vi "Transport Delay (DBL).vi"(2 "initialize":bool, 3 "delay":i32, 4 "reset":bool, 5 "input point":dbl format="%.2f") -> (1 "output point":dbl format="%.2f")   [LabVIEW 2020, in "NI_AdvCtrl_nonlinear.lvlib"]
doc: "LabVIEW no longer supports this VI. You can obtain similar functionality by installing the LabVIEW Simulation Module.\n\nStores input values with an arbitrarily long memory."
uses:
  <vilib>/addons/control/advanced/NI_AdvCtrl_nonlinear.lvlib
  <vilib>/addons/control/advanced/NI_AdvCtrl_continuous linear.lvlib
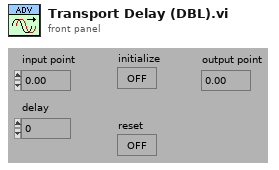
[diagram p1: front panel]
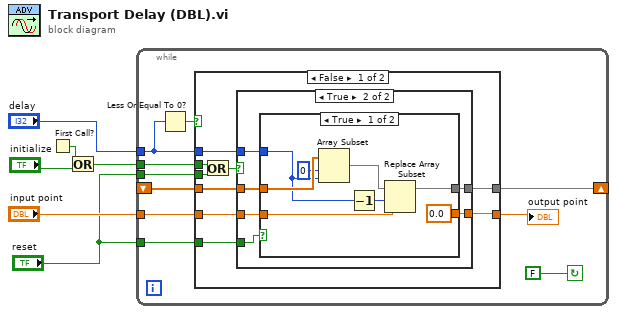
[diagram p0: block diagram]
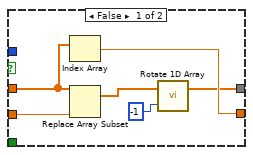
[diagram p2: hidden frame]
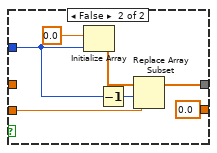
[diagram p3: hidden frame]
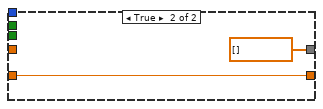
[diagram p4: hidden frame]
diagram:
  n1 = First Call?() -> (First Call?: T/F=w6:bool)
  n2 = Or(x=w6, y="initialize") -> (x .or. y?=w2:bool)
  n3 = while {
    tunnel: "input point" -> [w13]
    shift-left: _ -> [w14]
    shift-right: [w15] -> _
    tunnel: "delay" -> [w11]
    tunnel: w2 -> [w16]
    tunnel: "reset" -> [w8]
    tunnel: "reset" -> [w7]
    stop <- FALSE continue-if-true
    n4 = Less Or Equal To 0?(x=w11) -> (x <= 0?=w10:bool)
    n5 = case shown="False" w10 {
      tunnel: w16 -> [w25 _]
      tunnel: w11 -> [w24 _]
      tunnel: [w23 dbl[] []] -> w15
      tunnel: w14 -> [w22 _]
      tunnel: w13 -> [w21 w54]
      tunnel: [w20 w54] -> w9
      tunnel: w8 -> [w18 _]
      tunnel: w7 -> [w17 _]
      frame False {
        n6 = Or(x=w25, y=w18) -> (x .or. y?=w19:bool)
        n7 = case shown="True" w19 {
          tunnel: w24 -> [_ w35]
          tunnel: [w27 w37] -> w23
          tunnel: w22 -> [w30 w32]
          tunnel: w21 -> [w31 w36]
          tunnel: [w29 w34] -> w20
          tunnel: w17 -> [_ w33]
          frame False {
            n8 = Index Array(array=w30) -> (element=w29:dbl)  [unwired: 1 in]
            n9 = Replace Array Subset(array=w30, new element=w31) -> (w26:dbl[])  [unwired: 1 in]
            n10 = call <vilib>:"Rotate 1D Array.vi"("n"=-1, "array"=w26) -> ("array (last n elements first)"=w27:dbl[])  [unwired: 1 out]
          }
          frame True {
            n11 = case shown="True" w33 {
              tunnel: [w45 w50] -> w37
              tunnel: w36 -> [w44 w49]
              tunnel: w35 -> [w40 w48]
              tunnel: [0.0 ("input point") 0.0 ("input point")] -> w34
              tunnel: w32 -> [w41 _]
              frame True {
                n12 = Array Subset(array=w41, index=0, length=w40) -> (w38:dbl[])
                n13 = Decrement(x=w40) -> (x-1=w43:i32)
                n14 = Replace Array Subset(array=w38, new element=w44, index=w43) -> (w45:dbl[])
              }
              frame False {
                n15 = Initialize Array(0.0, w48) -> (w51:dbl[])
                n16 = Decrement(x=w48) -> (x-1=w47:i32)
                n17 = Replace Array Subset(array=w51, new element=w49, index=w47) -> (w50:dbl[])
              }
            }
          }
        }
      }
      frame True {
      }
    }
    "output point" <- w9
  }
